vi "binary_array.vi"(11 "Array":ext[](array[numeric])) -> (3 "binary array":ext[](array[numeric]))   [LabVIEW 2017]
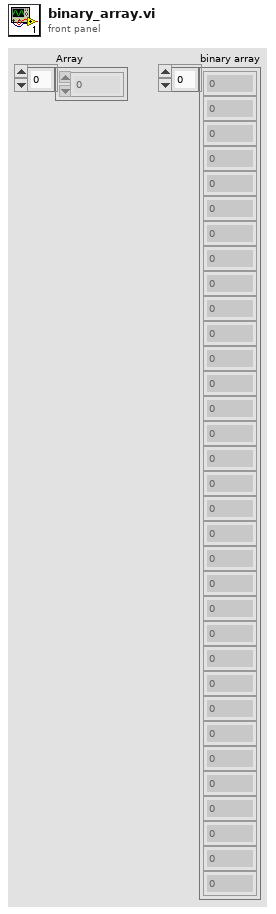
[diagram p1: front panel]
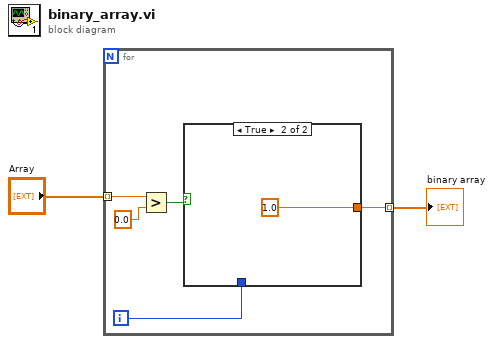
[diagram p0: block diagram]
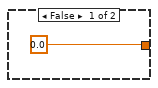
[diagram p2: hidden frame]
diagram:
  n1 = for {
    tunnel: "Array" -> [w6] mode=indexing
    tunnel: [w3] -> w1 mode=indexing
    i -> [w4]
    n2 = Greater?(x=w6, y=0.0) -> (0:w5:bool)
    n3 = case shown="True" w5 {
      tunnel: w4 -> [_ _]
      tunnel: [0.0 ("y") 1.0 ("y")] -> w3
      frame False {
      }
      frame True {
      }
    }
  }
  "binary array" <- w1
